vi "2[Scope] Set Sample Rate.vi"(11 "Frequency":dbl) -> (2 "Acquistion Time":dbl, 3 "Sample Rate":dbl)   [LabVIEW 2019]
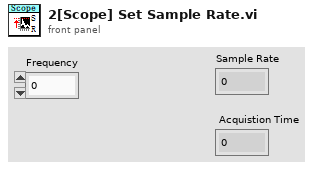
[diagram p1: front panel]
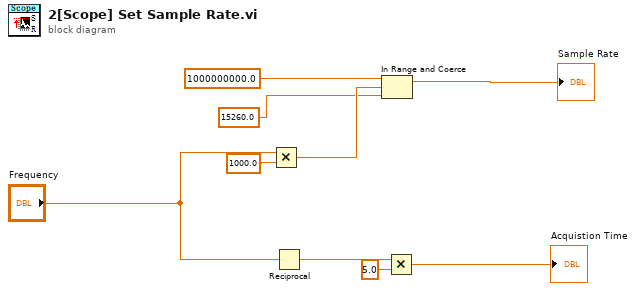
[diagram p0: block diagram]
diagram:
  n1 = Multiply(x="Frequency", y=1000.0) -> (x*y=w7:dbl)
  n2 = Reciprocal(x="Frequency") -> (1/x=w2:dbl)
  n3 = In Range and Coerce(upper limit=1000000000.0, x=w7, lower limit=15260.0) -> (coerced(x)=→"Sample Rate":dbl)  [unwired: 1 out]
  n4 = Multiply(x=w2, y=5.0) -> (x*y=→"Acquistion Time":dbl)
